vi "Result Engine Stop.vi"() -> (0 "error out":errorcluster)   [LabVIEW 2023, in "HardwareAbstractionLayer_LVOOP.lvlib" / "Report.lvclass"]
uses:
  Report.lvclass
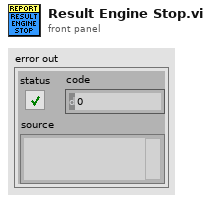
[diagram p1: front panel]
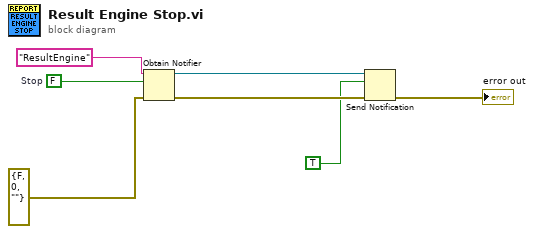
[diagram p0: block diagram]
diagram:
  w7 = FALSE  # Stop
  n1 = Obtain Notifier(name (unnamed)="ResultEngine", notification data type=w7, error in (no error)=errorcluster {"status"=FALSE, "code"=0, "source"=""}) -> (notifier out=w4:refnum<notifier>, error out=w3:errorcluster)  [unwired: 1 in, 1 out]
  n2 = Send Notification(notification=TRUE, notifier=w4, error in (no error)=w3) -> (error out=→"error out":errorcluster)  [unwired: 1 out]
